vi "Increment Timestamp.vi"(5 "Account for DST?":bool, 6 "Unit (second)":T1=enum."minute", 8 "Resolution (in selected unit)":dbl=1.0, 10 "timestamp (now)":timestamp) -> (3 "timestamp":timestamp)   [LabVIEW 2013]
doc: "Timestamp is not converted to UTC time, so the year being evaluated is the year of the timestamp, not the current year at GMT."
uses:
  Time Increment Units -- enum.ctl
  GregorianCal_MonthLengths.vi
  isLeapYear (integer).vi
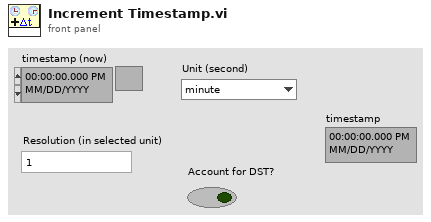
[diagram p1: front panel]
types:
  T1 = typedef "Time Increment Units -- enum.ctl" = enum16{"week", "day", "hour", "minute", "second", "millisecond", "microsecond", "nanosecond", "month", "year"}
  T2 = typedef "LVDateTimeRec.ctl" = cluster{"fractional second":dbl, "second":i32, "minute":i32, "hour":i32, "day of month":i32, "month":i32, "year":i32, "day of week":i32, "day of year":i32, "DST":i32}
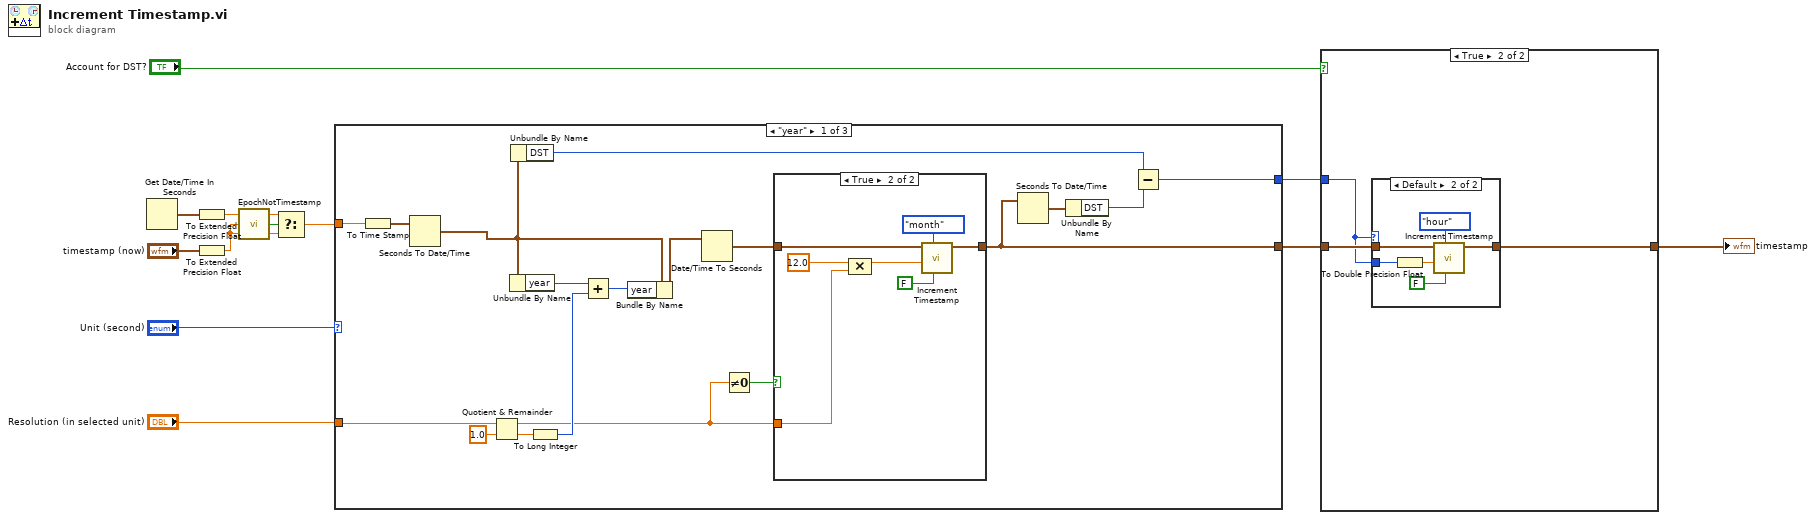
[diagram p0: block diagram]
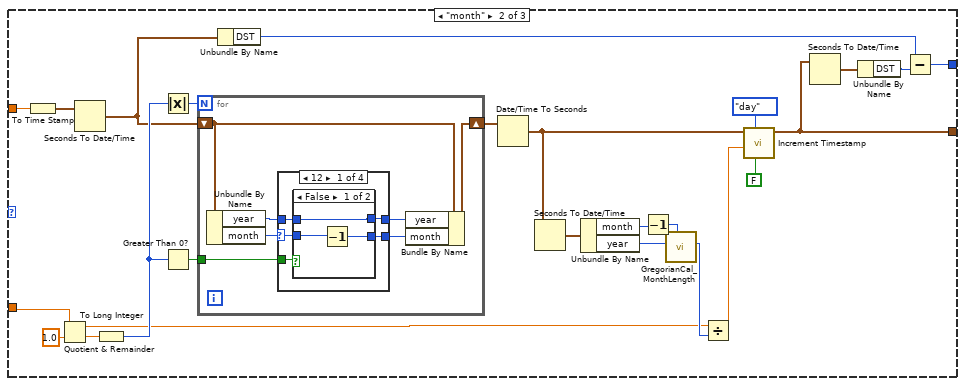
[diagram p5: hidden frame]
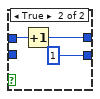
[diagram p6: hidden frame]
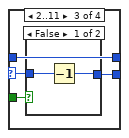
[diagram p8: hidden frame]
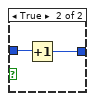
[diagram p9: hidden frame]
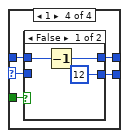
[diagram p10: hidden frame]
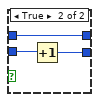
[diagram p11: hidden frame]
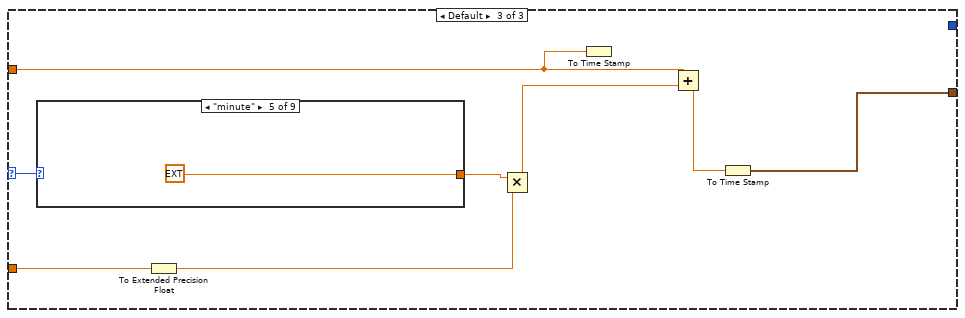
[diagram p12: hidden frame]
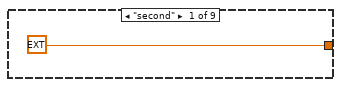
[diagram p13: hidden frame]
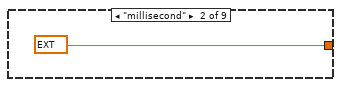
[diagram p14: hidden frame]
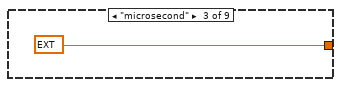
[diagram p15: hidden frame]
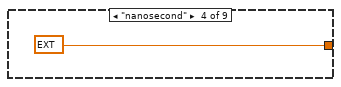
[diagram p16: hidden frame]
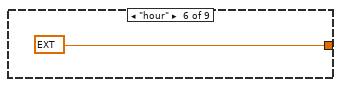
[diagram p17: hidden frame]
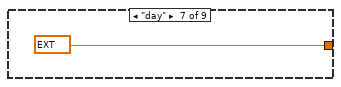
[diagram p18: hidden frame]
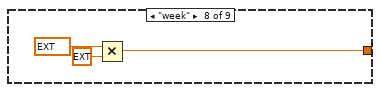
[diagram p19: hidden frame]
diagram:
  n1 = Get Date/Time In Seconds() -> (seconds since 1Jan1904=w11:timestamp)
  n2 = To Extended Precision Float(1:w11) -> (0:w10:ext)
  n3 = To Extended Precision Float(1:"timestamp (now)") -> (0:w9:ext)
  n4 = call "EpochNotTimestamp.vi"("Epoch Time"=w9) -> ("Not a Timestamp?"=w12:bool)  [unwired: 8 in]
  n5 = Select(t=w10, s=w12, f=w9) -> (s? t:f=w5:ext)
  n6 = case shown="\"year\"" "Unit (second)" {
    selector: "Unit (second)" -> [_ _ w108]
    tunnel: "Resolution (in selected unit)" -> [w27 w50 w110]
    tunnel: w5 -> [w14 w41 w103]
    tunnel: [w19 w42 w105] -> w3
    tunnel: [w16 w43 _] -> w1
    frame "year" {
      n7 = To Time Stamp(1:w14) -> (0:w15:timestamp)
      n8 = Seconds To Date/Time(time stamp (now)=w15) -> (date time rec=w13:T2)  [unwired: 1 in]
      n9 = Quotient & Remainder(x=w27, y=1.0) -> (x-y*floor(x/y)=w22:dbl, floor(x/y)=w26:dbl)
      n10 = Unbundle By Name(w13) -> ("year"=w30:i32)
      n11 = Unbundle By Name(w13) -> ("DST"=w18:i32)
      n12 = To Long Integer(number=w26) -> (32bit integer=w23:i32)
      n13 = Add(x=w30, y=w23) -> (x+y=w29:i32)
      n14 = Bundle By Name(cluster=w13, "year"=w29) -> (w21:T2)
      n15 = Date/Time To Seconds(2:w21) -> (0:w24:timestamp)  [unwired: 1 in]
      n16 = Not Equal To 0?(x=w22) -> (x != 0?=w25:bool)
      n17 = case shown="True" w25 {
        tunnel: w24 -> [w31 w38]
        tunnel: [w31 w33] -> w19
        tunnel: w22 -> [_ w35]
        frame False {
        }
        frame True {
          n18 = Compound Arithmetic op=MULTIPLY(12.0 ("x"), w35) -> (w34:dbl)
          n19 = call "Increment Timestamp.vi"("Account for DST?"=FALSE, "Unit (second)"=Time_Increment_Units_--_enum."month", "Resolution (in selected unit)"=w34, "timestamp (now)"=w38) -> ("timestamp"=w33:timestamp)  [unwired: 6 in]
        }
      }
      n20 = Seconds To Date/Time(time stamp (now)=w19) -> (date time rec=w20:T2)  [unwired: 1 in]
      n21 = Unbundle By Name(w20) -> ("DST"=w17:i32)
      n22 = Subtract(x=w18, y=w17) -> (x-y=w16:i32)
    }
    frame "month" {
      n23 = To Time Stamp(1:w41) -> (0:w40:timestamp)
      n24 = Quotient & Remainder(x=w50, y=1.0) -> (x-y*floor(x/y)=w52:dbl, floor(x/y)=w62:dbl)
      n25 = Seconds To Date/Time(time stamp (now)=w40) -> (date time rec=w39:T2)  [unwired: 1 in]
      n26 = To Long Integer(number=w62) -> (32bit integer=w58:i32)
      n27 = Absolute Value(x=w58) -> (abs(x)=w57:i32)
      n28 = Greater Than 0?(x=w58) -> (x > 0?=w56:bool)
      n29 = for {
        N: w57 -> [_]
        shift-right: [w65] -> w60
        shift-left: w39 -> [w66]
        tunnel: w56 -> [w64]
        n30 = Unbundle By Name(w66) -> ("year"=w68:i32, "month"=w69:i32)
        n31 = case shown="12" w69 {
          selector: w69 -> [w72 w82 w86 w95]
          tunnel: [w75 w82 w87 w96] -> w70
          tunnel: w68 -> [w74 w83 w85 w92]
          tunnel: [w73 w83 w85 w93] -> w67
          tunnel: w64 -> [w71 _ w84 w94]
          frame 12 {
            n32 = case shown="False" w71 {
              tunnel: [w77 1] -> w75
              tunnel: w74 -> [w78 w80]
              tunnel: [w78 w79] -> w73
              tunnel: w72 -> [w76 _]
              frame False {
                n33 = Decrement(x=w76) -> (x-1=w77:i32)
              }
              frame True {
                n34 = Increment(x=w80) -> (x+1=w79:i32)
              }
            }
          }
          frame Default {
          }
          frame 2..11 {
            n35 = case shown="False" w84 {
              tunnel: [w88 w91] -> w87
              tunnel: w86 -> [w89 w90]
              frame False {
                n36 = Decrement(x=w89) -> (x-1=w88:i32)
              }
              frame True {
                n37 = Increment(x=w90) -> (x+1=w91:i32)
              }
            }
          }
          frame 1 {
            n38 = case shown="False" w94 {
              tunnel: [12 w102] -> w96
              tunnel: w95 -> [_ w101]
              tunnel: [w97 w100] -> w93
              tunnel: w92 -> [w98 w100]
              frame False {
                n39 = Decrement(x=w98) -> (x-1=w97:i32)
              }
              frame True {
                n40 = Increment(x=w101) -> (x+1=w102:i32)
              }
            }
          }
        }
        n41 = Bundle By Name(cluster=w66, "year"=w67, "month"=w70) -> (w65:T2)
      }
      n42 = Unbundle By Name(w39) -> ("DST"=w45:i32)
      n43 = Date/Time To Seconds(2:w60) -> (0:w49:timestamp)  [unwired: 1 in]
      n44 = Seconds To Date/Time(time stamp (now)=w49) -> (date time rec=w59:T2)  [unwired: 1 in]
      n45 = Unbundle By Name(w59) -> ("month"=w48:i32, "year"=w55:i32)
      n46 = Decrement(x=w48) -> (x-1=w54:i32)
      n47 = call "GregorianCal_MonthLength.vi"("Month"=w54, "Year (0: this year)"=w55) -> ("Nb Days"=w53:i32)  [unwired: 9 in]
      n48 = Divide(x=w52, y=w53) -> (x/y=w51:dbl)
      n49 = call "Increment Timestamp.vi"("Account for DST?"=FALSE, "Unit (second)"=Time_Increment_Units_--_enum."day", "Resolution (in selected unit)"=w51, "timestamp (now)"=w49) -> ("timestamp"=w42:timestamp)  [unwired: 6 in]
      n50 = Seconds To Date/Time(time stamp (now)=w42) -> (date time rec=w46:T2)  [unwired: 1 in]
      n51 = Unbundle By Name(w46) -> ("DST"=w44:i32)
      n52 = Subtract(x=w45, y=w44) -> (x-y=w43:i32)
    }
    frame Default {
      n53 = case shown="\"minute\"" w108 {
        tunnel: [ext 1.0 ext 0.00099999999999999999996 ext 0.00000100000000000000000004 ext 1e-9 ext 60.0 ext 3600.0 ext 86400.0 w118 _] -> w109
        frame "second" {
        }
        frame "millisecond" {
        }
        frame "microsecond" {
        }
        frame "nanosecond" {
        }
        frame "minute" {
        }
        frame "hour" {
        }
        frame "day" {
        }
        frame "week" {
          n54 = Multiply(x=ext 86400.0, y=ext 7.0) -> (x*y=w118:ext)
        }
        frame Default {
        }
      }
      n55 = To Extended Precision Float(1:w110) -> (0:w104:ext)
      n56 = Multiply(x=w109, y=w104) -> (x*y=w107:ext)
      n57 = To Time Stamp(1:w103) -> ()  [unwired: 1 out]
      n58 = Add(x=w103, y=w107) -> (x+y=w106:ext)
      n59 = To Time Stamp(1:w106) -> (0:w105:timestamp)
    }
  }
  n60 = case shown="True" "Account for DST?" {
    tunnel: [w121 w124] -> w4
    tunnel: w3 -> [w121 w123]
    tunnel: w1 -> [_ w122]
    frame False {
    }
    frame True {
      n61 = case shown="Default" w122 {
        tunnel: w122 -> [_ w129]
        tunnel: [w125 w128] -> w124
        tunnel: w123 -> [w125 w127]
        frame 0 {
        }
        frame Default {
          n62 = To Double Precision Float(number=w129) -> (double precision float=w131:dbl)
          n63 = call "Increment Timestamp.vi"("Account for DST?"=FALSE, "Unit (second)"=Time_Increment_Units_--_enum."hour", "Resolution (in selected unit)"=w131, "timestamp (now)"=w127) -> ("timestamp"=w128:timestamp)  [unwired: 6 in]
        }
      }
    }
  }
  "timestamp" <- w4
